vi "Differential Drive Odometry.vi"(6 "Reset":bool, 9 "Angle (degrees)":dbl, 10 "Right Distance":dbl, 11 "Left Distance":dbl) -> (3 "Pose":T1)   [LabVIEW 2019]
uses:
  Geometry/Typedef/Pose2d.ctl
  Geometry/Typedef/Translation2d.ctl
  Geometry/Typedef/Rotation2d.ctl
  <vilib>/Analysis/coordinate.llb/2D Cartesian Coordinate Rotation (Scalar).vi
  <vilib>/Analysis/NI_AALPro.lvlib
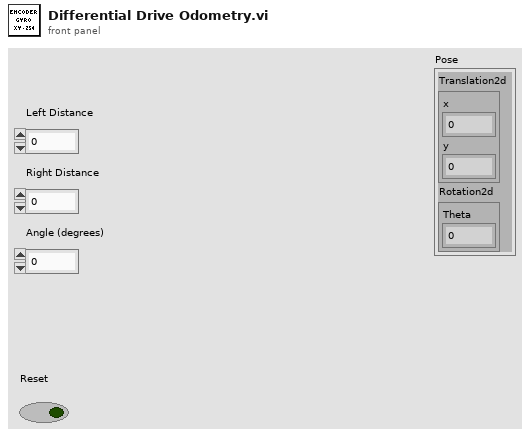
[diagram p1: front panel]
types:
  T1 = typedef "Pose2d.ctl" = cluster{"Translation2d":T2, "Rotation2d":T3}
  T2 = typedef "Translation2d.ctl" = cluster{"x":dbl, "y":dbl}
  T3 = typedef "Rotation2d.ctl" = cluster{"Theta":dbl}
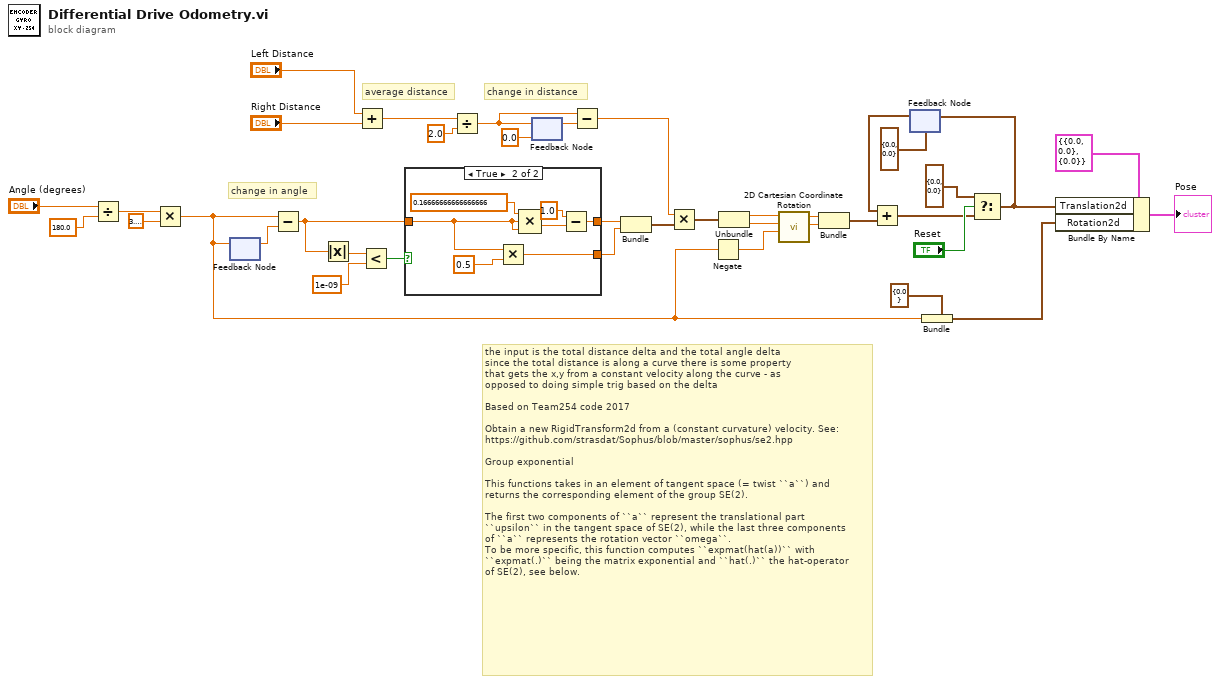
[diagram p0: block diagram]
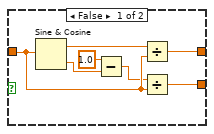
[diagram p2: hidden frame]
diagram:
  # "change in angle"
  # "the input is the total distance delta and the total angle delta\nsince the total distance is along a curve there is some property \nthat gets the x,y from a constant velocity along the curve - as\nopposed to doing simple trig based on the delta\n\nBased on Team254 code 2017\n\nObtain a new RigidTransform2d from a (constant curvature) velocity. See:\nhttps://github.com/strasdat/Sophus/blob/master/sophus/se2.hpp\n\nGroup exponential\n\nThis functions takes in an element of tangent space (= twist ``a``) and\nreturns the corresponding element of the group SE(2).\n\nThe first two components of ``a`` represent the translational part\n``upsilon`` in the tangent space of SE(2), while the last three components\nof ``a`` represents the rotation vector ``omega``.\nTo be more specific, this function computes ``expmat(hat(a))`` with\n``expmat(.)`` being the matrix exponential and ``hat(.)`` the hat-operator\nof SE(2), see below."
  # "change in distance"
  # "average distance"
  n1 = Divide(x="Angle (degrees)", y=180.0) -> (x/y=w11:dbl)
  n2 = Multiply(x=w11, y=3.141592653589793) -> (x*y=w1:dbl)
  n3 = feedback-in #1(w1) -> ()
  n4 = feedback #1() -> (w28:dbl)  [unwired: 1 in]
  n5 = Subtract(x=w1, y=w28) -> (x-y=w24:dbl)
  n6 = Absolute Value(x=w24) -> (abs(x)=w27:dbl)
  n7 = Add(x="Left Distance", y="Right Distance") -> (x+y=w33:dbl)
  n8 = Less?(x=w27, y=1e-09) -> (x < y?=w25:bool)
  n9 = case shown="True" w25 {
    tunnel: w24 -> [w44 w46]
    tunnel: [w40 w47] -> w23
    tunnel: [w39 w51] -> w22
    frame False {
      n10 = Sine & Cosine(0:w44) -> (1:w45:dbl, 2:w42:dbl)
      n11 = Subtract(x=1.0, y=w42) -> (x-y=w41:dbl)
      n12 = Divide(x=w45, y=w44) -> (x/y=w40:dbl)
      n13 = Divide(x=w41, y=w44) -> (x/y=w39:dbl)
    }
    frame True {
      n14 = Multiply(x=w46, y=0.5) -> (x*y=w51:dbl)
      n15 = Compound Arithmetic op=MULTIPLY(0.16666666666666666 ("y"), w46, w46) -> (w50:dbl)
      n16 = Subtract(x=1.0, y=w50) -> (x-y=w47:dbl)
    }
  }
  n17 = Divide(x=w33, y=2.0) -> (x/y=w32:dbl)
  n18 = feedback #2(0.0) -> (w38:dbl)
  n19 = feedback-in #2(w32) -> ()
  n20 = Subtract(x=w32, y=w38) -> (x-y=w20:dbl)
  n21 = Bundle(w23, w22) -> (w21:cluster{dbl, dbl})  [unwired: 1 in]
  n22 = Multiply(x=w20, y=w21) -> (x*y=w19:cluster{dbl, dbl})
  n23 = Negate(x=w1) -> (-x=w5:dbl)
  n24 = Unbundle(w19) -> (w18:dbl, w17:dbl)
  n25 = call-poly <vilib>:"2D Cartesian Coordinate Rotation.vi"("theta"=w5, "y"=w17, "x"=w18) -> ("y out"=w15:dbl, "x out"=w16:dbl)  [unwired: 6 in, 1 out]
  n26 = Bundle("x out"=w16, "y out"=w15) -> (w14:cluster{"x out":dbl, "y out":dbl})  [unwired: 1 in]
  n27 = feedback #3(T2 {"x"=0.0, "y"=0.0} ("Translation2d")) -> (w36:T2)
  n28 = Add(x=w36, y=w14) -> (x+y=w29:T2)
  n29 = Bundle(cluster=T3 {"Theta"=0.0} ("Rotation2d"), "Theta"=w1) -> (w3:T3)
  n30 = Select(t=T2 {"x"=0.0, "y"=0.0} ("Translation2d"), s="Reset", f=w29) -> (s? t:f=w6:T2)
  n31 = feedback-in #3(w6) -> ()
  n32 = Bundle By Name(cluster=T1 {"Translation2d"={"x"=0.0, "y"=0.0}, "Rotation2d"={"Theta"=0.0}} ("Pose2d"), "Translation2d"=w6, "Rotation2d"=w3) -> (→"Pose":T1)
